vi "Global.vi"() -> ()   [LabVIEW 2013]
panel:
  in  "Velocity Array":dbl[][](array[numeric])=[[0.7, 0.5], [0.1, 0.06]]
  out "Number of samples":i32
  in  "Deviation measurement additional range":dbl=0.05
  in  "Peak amplitude treshold":dbl=0.2
  in  "Interface Peak Left":refnum<vi>
  in  "Interface Peak Right Graph":refnum<vi>
  in  "Interface Coearse Peak Graph":refnum<vi>
  in  "Interface Progress Label":refnum<vi>
  in  "Interface Progress Bar":refnum<vi>
  in  "Measurement Iterations":u32=1
  in  "Coarse peak position":dbl
  in  "Callibration peak right":dbl
  in  "Callibration peak left":dbl
  in  "Fine Calibration Iterations":u32=1
  in  "Fine Calibration Range":dbl=0.05
  in  "Fine Callibration Velocity":dbl=0.05
  in  "Coarse Callibration Velocity":dbl=2.5
  in  "Rate":dbl=10000.0
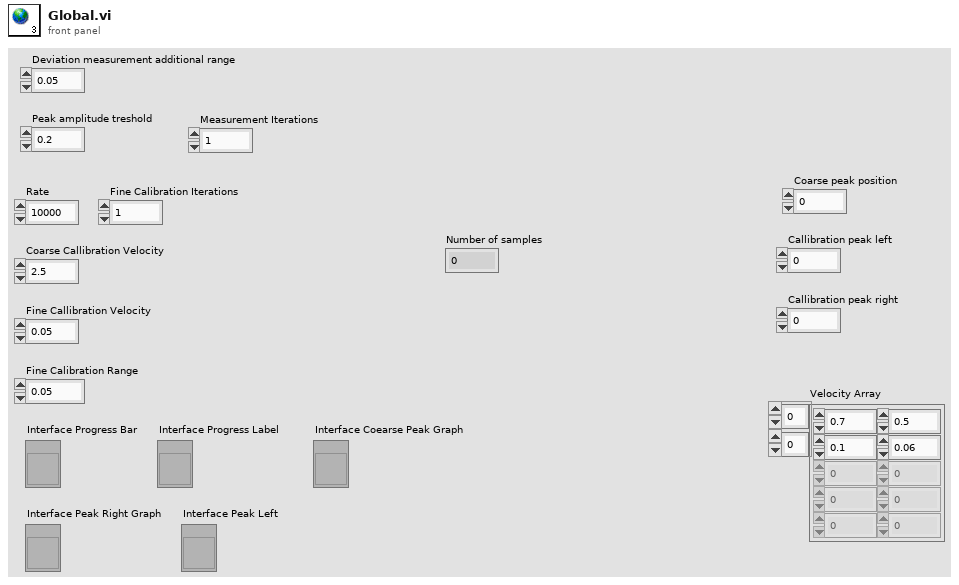
[diagram p1: front panel]
diagram:
